vi "ex_1.vi"() -> ()   [LabVIEW 2020]
panel:
  out "String":string
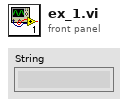
[diagram p1: front panel]
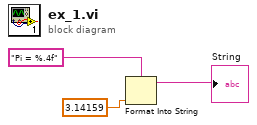
[diagram p0: block diagram]
diagram:
  n1 = Format Into String(format string="Pi = %.4f", 3.14159) -> (resulting string=→"String":string)  [unwired: 2 in, 1 out]
